vi "ReadAllCtlRefs_Core.vi"(8 "error in (no error)":errorcluster, 11 "CtlReferences in":refnum<class "CtlReferences.lvclass">) -> (0 "error out":errorcluster, 1 "Values":refnum<vi>[](array[refnum]), 2 "Names":string[](array[string]), 3 "CtlReferences out":refnum<class "CtlReferences.lvclass">)   [LabVIEW 2020, in "CtlReferences.lvlib" / "CtlReferences.lvclass"]
uses:
  CtlReferences.lvclass
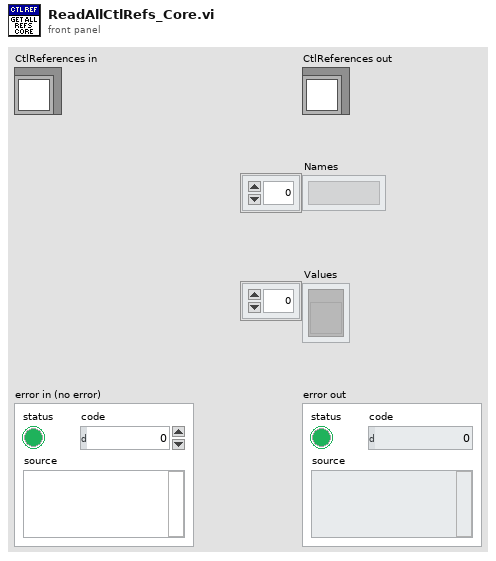
[diagram p1: front panel]
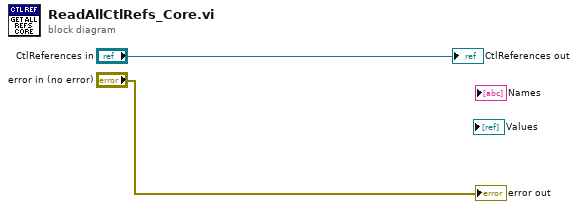
[diagram p0: block diagram]
diagram:
  "CtlReferences out" <- "CtlReferences in"
  "error out" <- "error in (no error)"
